vi "App_new_stream.vi"() -> ()   [LabVIEW 2015]
uses:
  <vilib>/DAQmx/read.llb/DAQmx Read (Analog Wfm 1Chan NSamp).vi
  <vilib>/DAQmx/miscellaneous.llb/DAQmx Fill In Error Info.vi
panel:
  in  "task out":refnum<k21>
  out "Button 2":u16
  out "Waveform Chart 2":waveform(dbl)
  out "Button":u16
  in  "Tab Control":T1(tab)
  out "min value":dbl
  out "max value":dbl
  out "Delta(s)":dbl
  in  "Zero":bool
  out "Average":dbl
  in  "mA/uA":bool
  out "Waveform Graph":waveform(dbl)(graph)
  in  "uA/mA":bool=TRUE
  out "Waveform Graph 2":waveform(dbl)(graph)
  out "Average (uA)":dbl
  in  "PAUSE":bool
  out "Vbat":dbl
  out "Waveform Chart":dbl(graph)
  in  "Number of samples uC Board":i32=10000
  in  "USB DAQ":tag="Dev1"
  out "Waveform Chart 3":dbl(graph)
  in  "file List":i32(listbox)
  out "2D Picture":picture
  # "FW Validation - Current Tracking V1.0"
  # "For uC Board: 20kS/s"
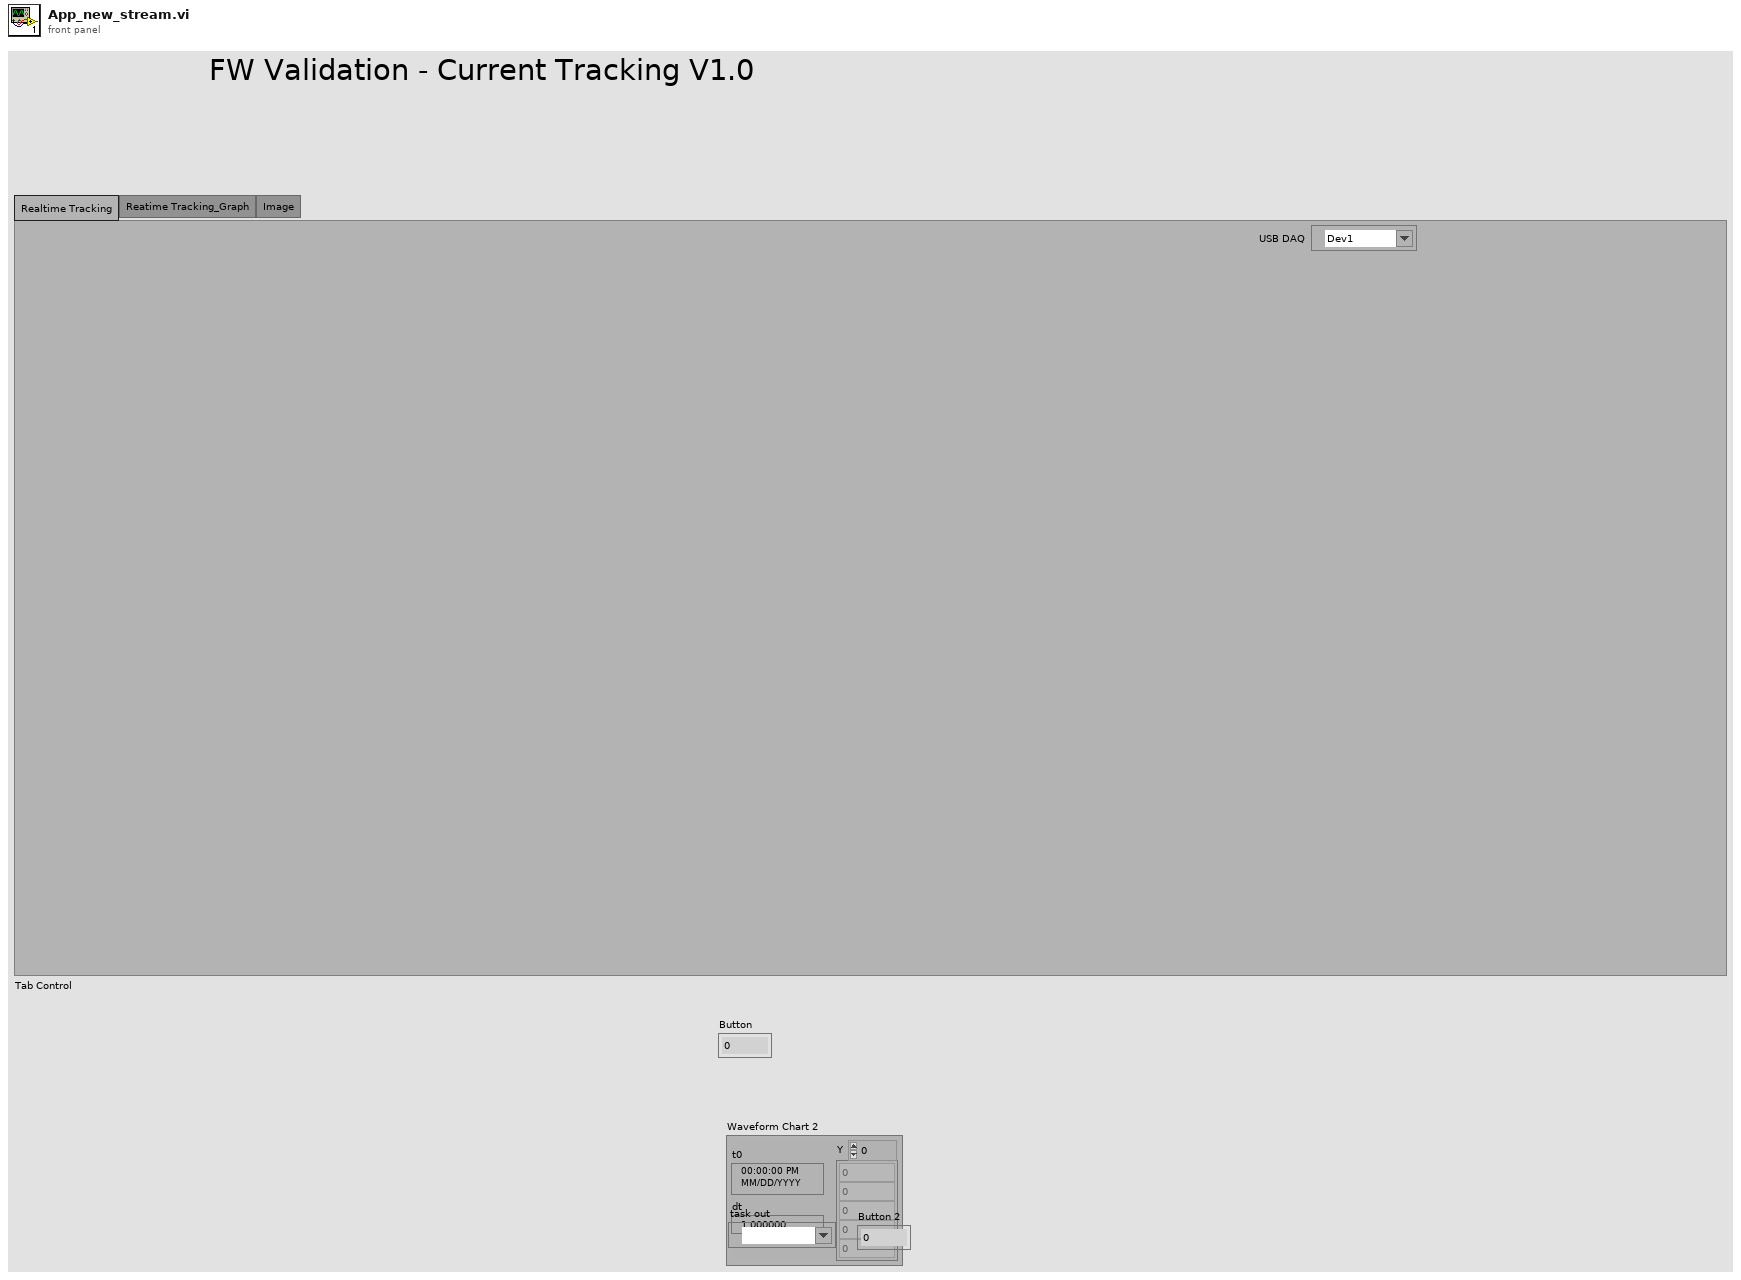
[diagram p1: front panel]
types:
  T1 = enum32{"Realtime Tracking", "Reatime Tracking_Graph", "Image"}
  T2 = typedef "imagedata.ctl" = cluster{"image type":i32, "image depth":i32, "image":u8[], "mask":u8[], "colors":u32[], "Rectangle":cluster{"left":i16, "top":i16, "right":i16, "bottom":i16}}
  T3 = typedef "LVCursorListTypeDef.ctl" = cluster{"Name":string, "Color":u32, "Style":u8, "Point Style":u8, "Name Visible":bool, "Allow Drag":bool, "Cursor Mode":u32, "Plot":i32, "Index":i32, "Position":cluster{"X":dbl, "Y":dbl}, "X Scale":u32, "Y Scale":u32, "Watch Plots":i32[], "Watch All Plots":bool, "Plot Area":i32, "Label Offset":cluster{"X":dbl, "Y":dbl}}[]
  T4 = cluster{"Name":string, "Color":u32, "Style":u8, "Point Style":u8, "Name Visible":bool, "Allow Drag":bool, "Cursor Mode":u32, "Plot":i32, "Index":i32, "Position":cluster{"X":dbl, "Y":dbl}, "X Scale":u32, "Y Scale":u32, "Watch Plots":i32[], "Watch All Plots":bool, "Plot Area":i32, "Label Offset":cluster{"X":dbl, "Y":dbl}}
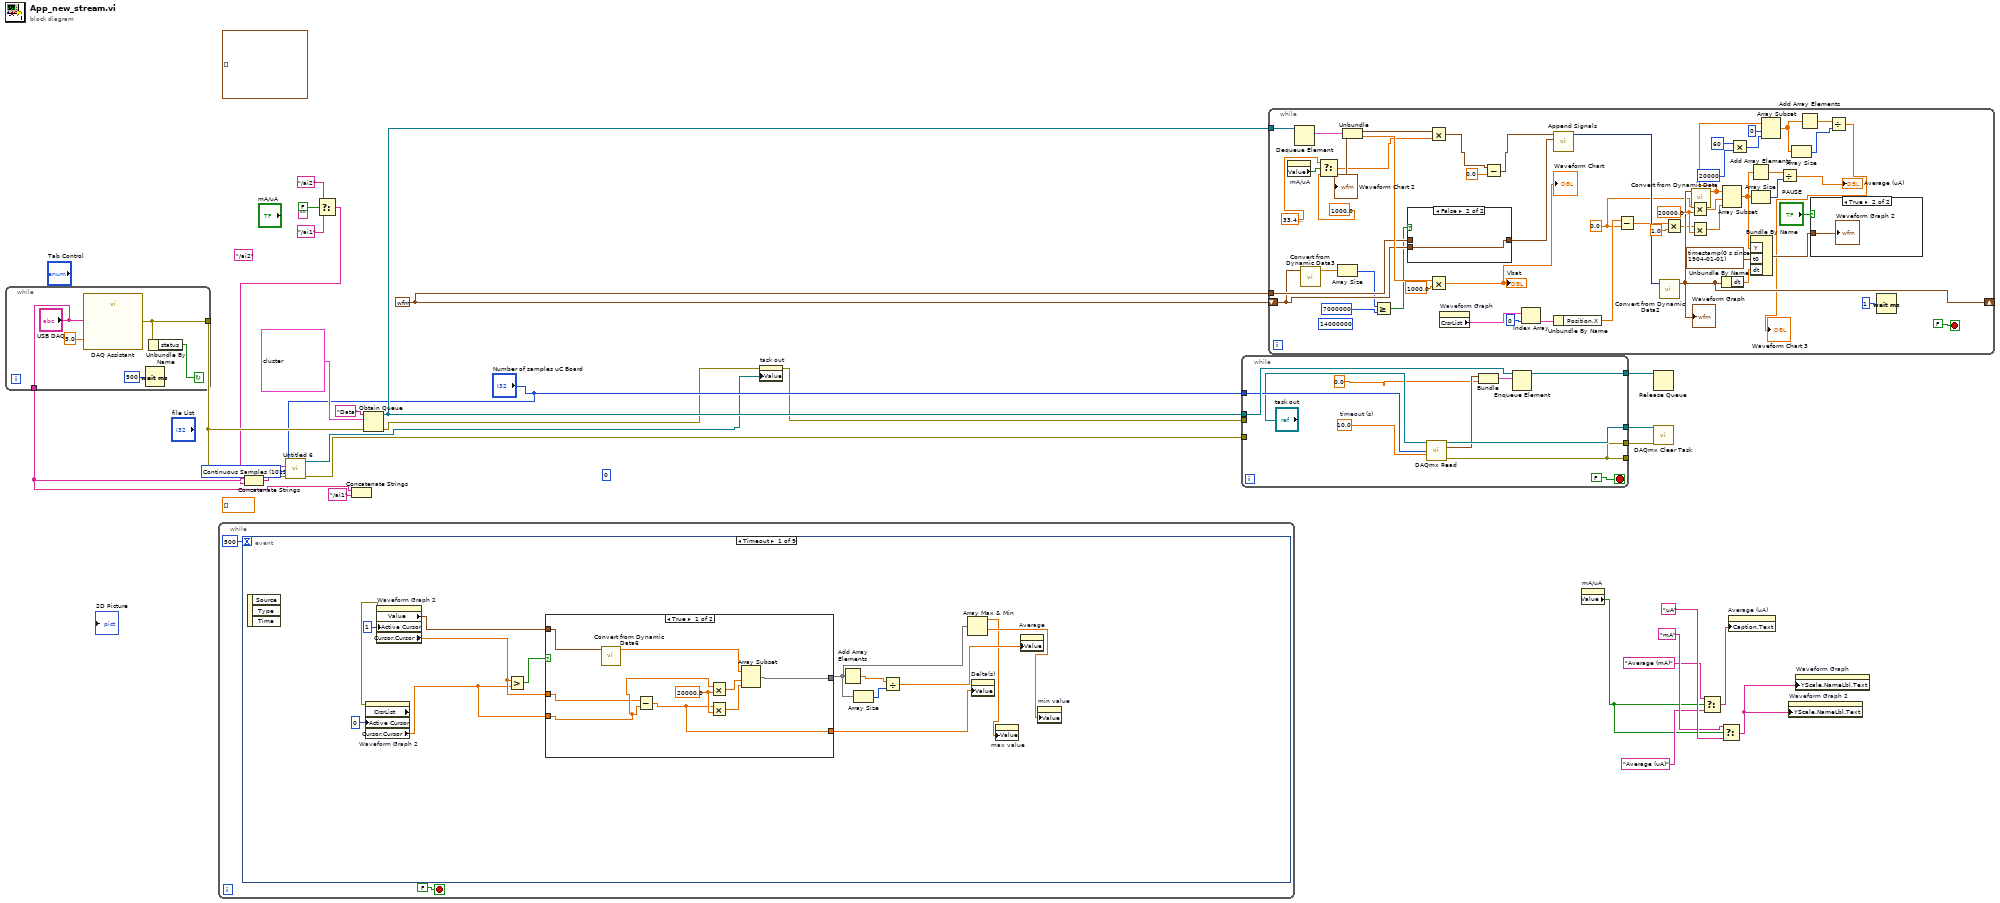
[diagram p0: block diagram]
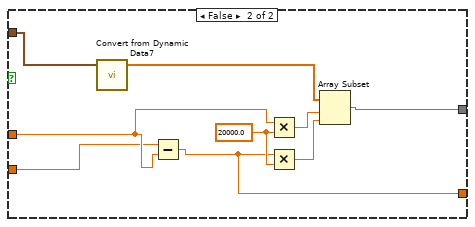
[diagram p2: hidden frame]
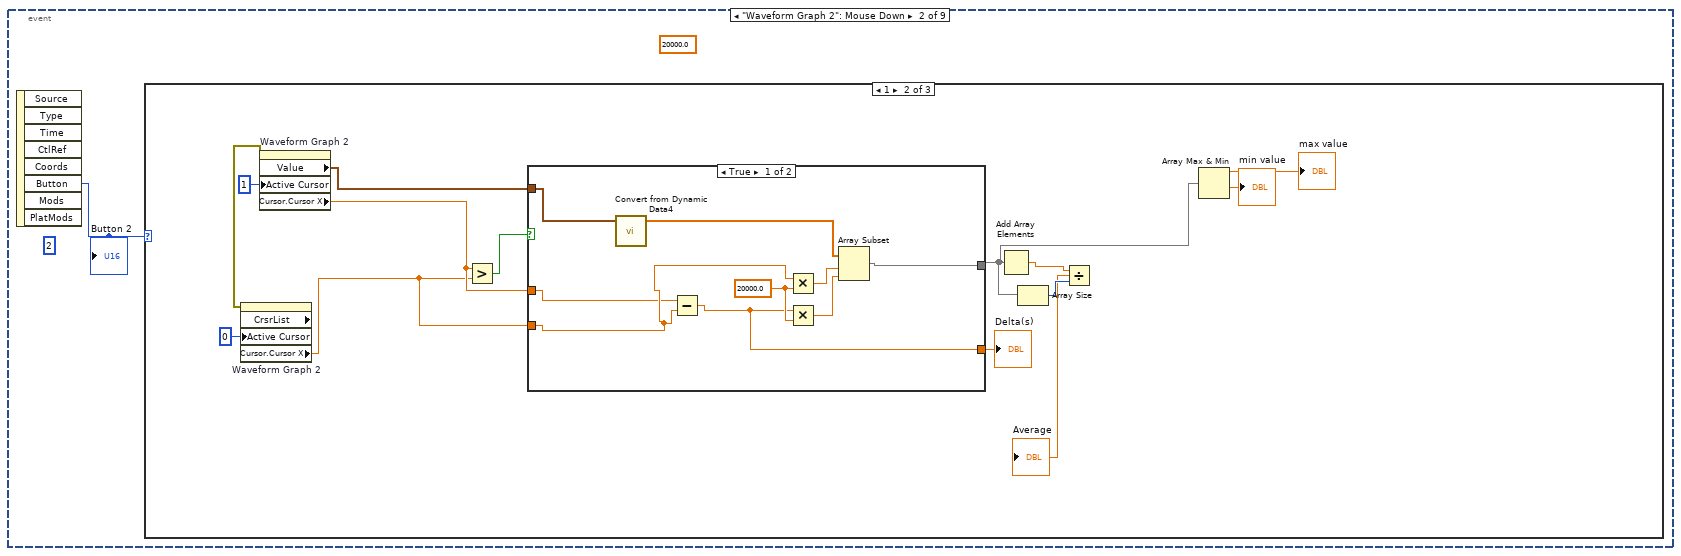
[diagram p3: hidden frame]
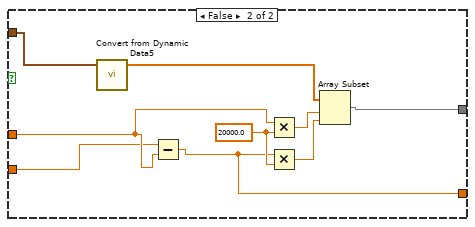
[diagram p5: hidden frame]
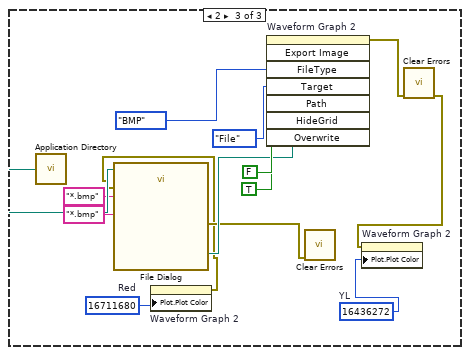
[diagram p6: hidden frame]
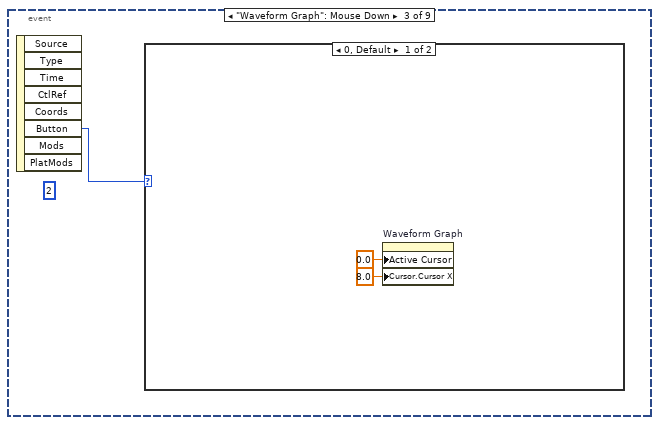
[diagram p7: hidden frame]
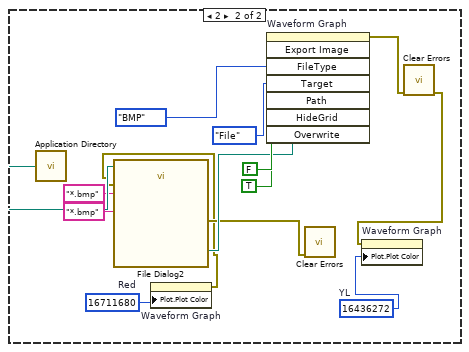
[diagram p8: hidden frame]
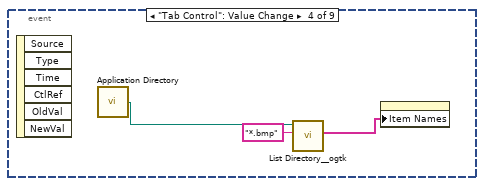
[diagram p9: hidden frame]
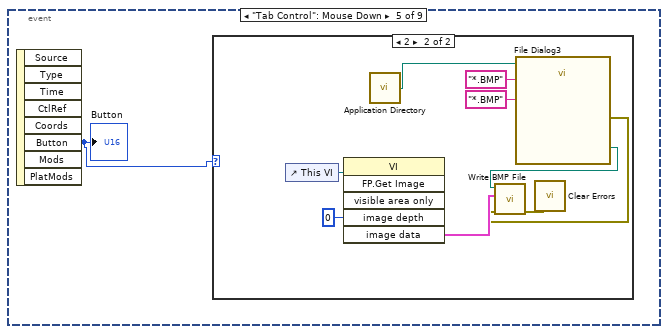
[diagram p10: hidden frame]
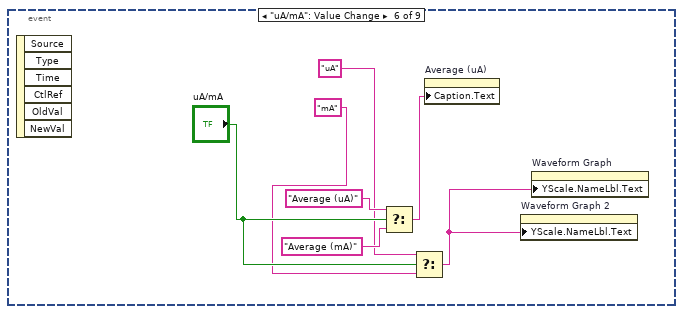
[diagram p12: hidden frame]
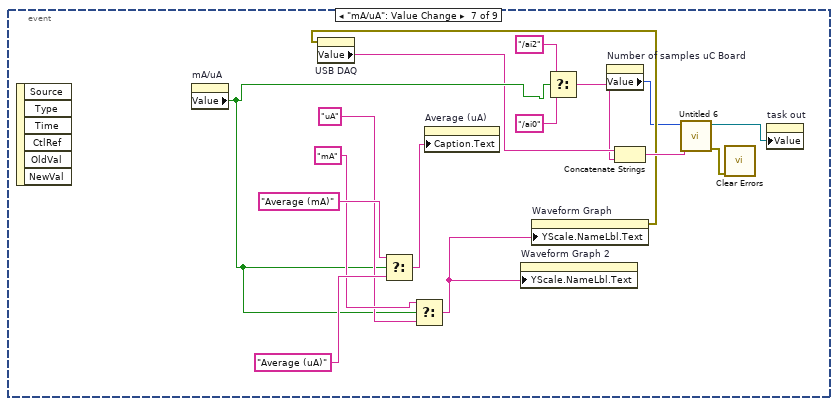
[diagram p13: hidden frame]
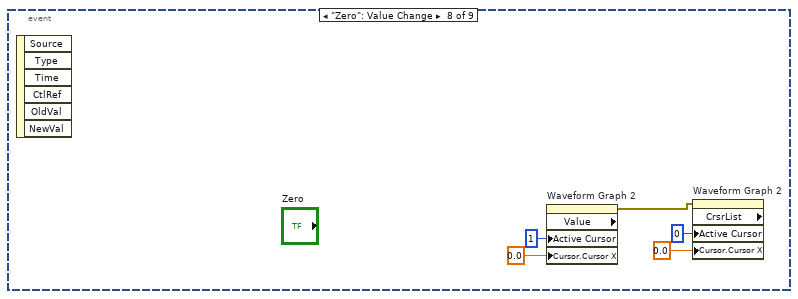
[diagram p14: hidden frame]
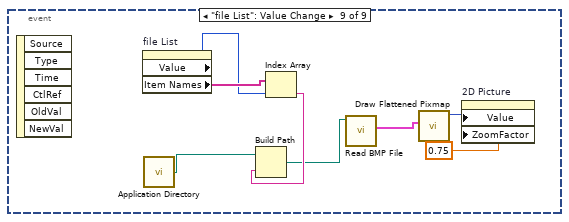
[diagram p15: hidden frame]
diagram:
  (unwired) "" ("f")
  w2 = 10123 items=["Finite Samples"=10178, "Continuous Samples"=10123, "Hardware Timed Single Point"=12522] ("sample mode")
  (unwired) u32 0 ("Active Cursor")
  (unwired) "/ai2" ("string")
  w20 = waveform(dbl) {"t0"=timestamp(0 s since 1904-01-01), "dt"=0.0, "Y"=[]} ("data")
  (unwired) waveform(dbl)[] [] ("History Data")
  (unwired) dbl[] [] ("Array")
  n1 = while {
    tunnel: [w31] -> w23
    tunnel: ["USB DAQ"] -> w17
    stop <- w30 continue-if-true
    n2 = call "DAQ Assistant"("data"=5.0, "device name"="USB DAQ") -> ("error out"=w31:errorcluster)  [unwired: 16 in, 1 out]
    n3 = Wait (ms)(milliseconds to wait=u32 500) -> ()  [unwired: 1 out]
    n4 = Unbundle By Name(w31) -> ("status"=w30:bool)
  }
  n5 = while {
    stop <- FALSE stop-if-true
    n6 = event shown="[0] Timeout" {
      selector: _ -> [_ _ _ _ _ _ _ _ _]
      dyn-events: _ -> [_ _ _ _ _ _ _ _ _]
      timeout: 500 -> [_ _ _ _ _ _ _ _ _]
      event Timeout {
        n7 = event-data() -> ()  [unwired: 1 in, 3 out]
        n8 = property on="Waveform Graph 2" class="WFGraph (strict)"("Active Cursor"=u32 1) -> (error out=w44:errorcluster, "Value"=w40:waveform(dbl), "Cursor.Cursor X"=w46:dbl)  [unwired: 2 in, 1 out]
        n9 = property on="Waveform Graph 2" class="WFGraph (strict)" props=["CrsrList", "Active Cursor", "Cursor", "Cursor X"](error in=w44, "Active Cursor"=u32 0) -> ("Cursor.Cursor X"=w45:dbl)  [unwired: 1 in, 3 out]
        n10 = Greater?(x=w46, y=w45) -> (0:w47:bool)
        n11 = case shown="True" w47 {
          tunnel: w40 -> [w58 w67]
          tunnel: w46 -> [w51 w61]
          tunnel: w45 -> [w52 w60]
          tunnel: [w53 w62] -> w41
          tunnel: [w50 w59] -> w39
          frame True {
            w56 = 20000.0 ("y")
            n12 = call "Convert from Dynamic Data6"("Dynamic Data Type"=w58) -> ("Array"=w54:dbl[])  [unwired: 3 in]
            n13 = Subtract(x=w51, y=w52) -> (x-y=w50:dbl)
            n14 = Multiply(x=w52, y=w56) -> (x*y=w57:dbl)
            n15 = Multiply(x=w50, y=w56) -> (x*y=w55:dbl)
            n16 = Array Subset(array=w54, index=w57, length=w55) -> (w53:dbl[])
          }
          frame False {
            w65 = 20000.0 ("y")
            n17 = call "Convert from Dynamic Data7"("Dynamic Data Type"=w67) -> ("Array"=w63:dbl[])  [unwired: 3 in]
            n18 = Subtract(x=w60, y=w61) -> (x-y=w59:dbl)
            n19 = Multiply(x=w61, y=w65) -> (x*y=w66:dbl)
            n20 = Multiply(x=w59, y=w65) -> (x*y=w64:dbl)
            n21 = Array Subset(array=w63, index=w66, length=w64) -> (w62:dbl[])
          }
        }
        n22 = Add Array Elements(numeric array=w41) -> (sum=w43:dbl)
        n23 = Array Size(array=w41) -> (size(s)=w42:i32)
        n24 = Divide(x=w43, y=w42) -> (x/y=w38:dbl)
        n25 = Array Max & Min(array=w41) -> (max value=w36:dbl, min value=w37:dbl)  [unwired: 2 out]
        n26 = property on="Delta(s)" class="DigNum (strict)"("Value"=w39) -> ()  [unwired: 2 in, 2 out]
        n27 = property on="max value" class="DigNum (strict)"("Value"=w36) -> ()  [unwired: 2 in, 2 out]
        n28 = property on="Average" class="DigNum (strict)"("Value"=w38) -> ()  [unwired: 2 in, 2 out]
        n29 = property on="min value" class="DigNum (strict)"("Value"=w37) -> ()  [unwired: 2 in, 2 out]
      }
      event "Waveform Graph 2": Mouse Down {
        (unwired) 20000.0 ("y")
        (unwired) u16 2 ("Button")
        n30 = event-data() -> ("Button"=w68:u16)  [unwired: 1 in, 7 out]
        "Button 2" <- w68
        n31 = case shown="1" w68 {
          frame 0, Default {
          }
          frame 1 {
            n32 = property on="Waveform Graph 2" class="WFGraph (strict)"("Active Cursor"=u32 1) -> (error out=w77:errorcluster, "Value"=w69:waveform(dbl), "Cursor.Cursor X"=w79:dbl)  [unwired: 2 in, 1 out]
            n33 = property on="Waveform Graph 2" class="WFGraph (strict)" props=["CrsrList", "Active Cursor", "Cursor", "Cursor X"](error in=w77, "Active Cursor"=u32 0) -> ("Cursor.Cursor X"=w78:dbl)  [unwired: 1 in, 3 out]
            n34 = Greater?(x=w79, y=w78) -> (0:w80:bool)
            n35 = case shown="True" w80 {
              tunnel: w69 -> [w91 w100]
              tunnel: w79 -> [w84 w94]
              tunnel: w78 -> [w85 w93]
              tunnel: [w86 w95] -> w72
              tunnel: [w83 w92] -> w73
              frame True {
                w89 = 20000.0 ("y")
                n36 = call "Convert from Dynamic Data4"("Dynamic Data Type"=w91) -> ("Array"=w87:dbl[])  [unwired: 3 in]
                n37 = Subtract(x=w84, y=w85) -> (x-y=w83:dbl)
                n38 = Multiply(x=w85, y=w89) -> (x*y=w90:dbl)
                n39 = Multiply(x=w83, y=w89) -> (x*y=w88:dbl)
                n40 = Array Subset(array=w87, index=w90, length=w88) -> (w86:dbl[])
              }
              frame False {
                w98 = 20000.0 ("y")
                n41 = call "Convert from Dynamic Data5"("Dynamic Data Type"=w100) -> ("Array"=w96:dbl[])  [unwired: 3 in]
                n42 = Subtract(x=w93, y=w94) -> (x-y=w92:dbl)
                n43 = Multiply(x=w94, y=w98) -> (x*y=w99:dbl)
                n44 = Multiply(x=w92, y=w98) -> (x*y=w97:dbl)
                n45 = Array Subset(array=w96, index=w99, length=w97) -> (w95:dbl[])
              }
            }
            "Delta(s)" <- w73
            n46 = Add Array Elements(numeric array=w72) -> (sum=w76:dbl)
            n47 = Array Size(array=w72) -> (size(s)=w75:i32)
            n48 = Divide(x=w76, y=w75) -> (x/y=→"Average":dbl)
            n49 = Array Max & Min(array=w72) -> (max value=→"max value":dbl, min value=→"min value":dbl)  [unwired: 2 out]
          }
          frame 2 {
            w101 = u32 16436272  # YL
            w103 = u32 16711680  # Red
            n50 = call <vilib>:"Application Directory.vi"() -> ("Application Directory"=w110:path)
            n51 = property on="Waveform Graph 2" class="WFGraph (strict)"("Plot.Plot Color"=w103) -> (error out=w104:errorcluster)  [unwired: 2 in, 1 out]
            n52 = call "File Dialog"("start path"=w110, "error in"=w104, "pattern (all files)"="*.bmp", "pattern label"="*.bmp") -> ("selected path"=w107:path, "error out"=w106:errorcluster)  [unwired: 8 in, 2 out]
            n53 = invoke on="Waveform Graph 2" class="WFGraph (strict)" method="Export Image"("FileType"=enum32{"BMP", "EPS", "EMF", "PICT"}."BMP" ("File Type"), "Target"=enum32{"File", "Clipboard"}."File", "Path"=w107, "HideGrid"=FALSE ("Hide Grid"), "Overwrite"=TRUE ("Always Overwrite")) -> (error out=w105:errorcluster)  [unwired: 3 in, 7 out]
            n54 = call <vilib>:"Clear Errors.vi"("error in (no error)"=w106) -> ()  [unwired: 5 in, 2 out]
            n55 = call <vilib>:"Clear Errors.vi"("error in (no error)"=w105) -> ("error out"=w102:errorcluster)  [unwired: 5 in, 1 out]
            n56 = property on="Waveform Graph 2" class="WFGraph (strict)"(error in=w102, "Plot.Plot Color"=w101) -> ()  [unwired: 1 in, 2 out]
          }
        }
      }
      event "Waveform Graph": Mouse Down {
        (unwired) u16 2 ("Button")
        n57 = event-data() -> ("Button"=w115:u16)  [unwired: 1 in, 7 out]
        n58 = case shown="0, Default" w115 {
          frame 0, Default {
            n59 = property on="Waveform Graph" class="WFGraph (strict)"("Active Cursor"=0.0 ("Cursor.Cursor Position:Cursor X"), "Cursor.Cursor X"=8.0 ("Cursor.Cursor Position:Cursor X")) -> ()  [unwired: 2 in, 2 out]
          }
          frame 2 {
            w118 = u32 16436272  # YL
            w120 = u32 16711680  # Red
            n60 = call <vilib>:"Application Directory.vi"() -> ("Application Directory"=w127:path)
            n61 = property on="Waveform Graph" class="WFGraph (strict)"("Plot.Plot Color"=w120) -> (error out=w121:errorcluster)  [unwired: 2 in, 1 out]
            n62 = call "File Dialog2"("start path"=w127, "error in"=w121, "pattern (all files)"="*.bmp", "pattern label"="*.bmp") -> ("selected path"=w124:path, "error out"=w123:errorcluster)  [unwired: 8 in, 2 out]
            n63 = invoke on="Waveform Graph" class="WFGraph (strict)" method="Export Image"("FileType"=enum32{"BMP", "EPS", "EMF", "PICT"}."BMP" ("File Type"), "Target"=enum32{"File", "Clipboard"}."File", "Path"=w124, "HideGrid"=FALSE ("Hide Grid"), "Overwrite"=TRUE ("Always Overwrite")) -> (error out=w122:errorcluster)  [unwired: 3 in, 7 out]
            n64 = call <vilib>:"Clear Errors.vi"("error in (no error)"=w123) -> ()  [unwired: 5 in, 2 out]
            n65 = call <vilib>:"Clear Errors.vi"("error in (no error)"=w122) -> ("error out"=w119:errorcluster)  [unwired: 5 in, 1 out]
            n66 = property on="Waveform Graph" class="WFGraph (strict)"(error in=w119, "Plot.Plot Color"=w118) -> ()  [unwired: 1 in, 2 out]
          }
        }
      }
      event "Tab Control": Value Change {
        n67 = event-data() -> ()  [unwired: 1 in, 6 out]
        n68 = call <vilib>:"Application Directory.vi"() -> ("Application Directory"=w134:path)
        n69 = call <userlib>:"List Directory__ogtk.vi"("pattern"="*.bmp", "directory path"=w134) -> ("file names"=w132:string[])  [unwired: 2 in, 3 out]
        n70 = property on="file List" class="LstBox (strict)"("Item Names"=w132) -> ()  [unwired: 2 in, 2 out]
      }
      event "Tab Control": Mouse Down {
        n71 = event-data() -> ("Button"=w135:u16)  [unwired: 1 in, 7 out]
        "Button" <- w135
        n72 = case shown="2" w135 {
          frame 0, Default {
          }
          frame 2 {
            n73 = control-ref of="This VI"() -> (w144:refnum<vi>)
            n74 = invoke class="VI" method="FP.Get Image"(reference=w144, "image depth"=0 ("Image Depth")) -> ("image data"=w142:T2)  [unwired: 4 in, 5 out]
            n75 = call <vilib>:"Application Directory.vi"() -> ("Application Directory"=w138:path)
            n76 = call "File Dialog3"("start path"=w138, "pattern (all files)"="*.BMP", "pattern label"="*.BMP") -> ("selected path"=w141:path, "error out"=w140:errorcluster)  [unwired: 9 in, 2 out]
            n77 = call <vilib>:"Write BMP File.vi"("error in (no error)"=w140, "image data"=w142, "path to BMP file"=w141) -> ("error out"=w136:errorcluster)  [unwired: 7 in, 1 out]
            n78 = call <vilib>:"Clear Errors.vi"("error in (no error)"=w136) -> ()  [unwired: 5 in, 2 out]
          }
        }
      }
      event "uA/mA": Value Change {
        n79 = event-data() -> ()  [unwired: 1 in, 6 out]
        n80 = Select(t="Average (uA)" ("Caption.Text"), s="uA/mA", f="Average (mA)" ("Caption.Text")) -> (s? t:f=w151:string)
        n81 = Select(t="uA" ("Caption.Text"), s="uA/mA", f="mA" ("Caption.Text")) -> (s? t:f=w145:string)
        n82 = property on="Average (uA)" class="DigNum (strict)"("Caption.Text"=w151) -> ()  [unwired: 2 in, 2 out]
        n83 = property on="Waveform Graph 2" class="WFGraph (strict)"("YScale.NameLbl.Text"=w145) -> ()  [unwired: 2 in, 2 out]
        n84 = property on="Waveform Graph" class="WFGraph (strict)"("YScale.NameLbl.Text"=w145) -> ()  [unwired: 2 in, 2 out]
      }
      event "mA/uA": Value Change {
        n85 = event-data() -> ()  [unwired: 1 in, 6 out]
        n86 = property on="mA/uA" class="Bool (strict)"() -> ("Value"=w159:bool)  [unwired: 2 in, 2 out]
        n87 = Select(t="Average (mA)" ("Caption.Text"), s=w159, f="Average (uA)" ("Caption.Text")) -> (s? t:f=w167:string)
        n88 = Select(t="mA" ("Caption.Text"), s=w159, f="uA" ("Caption.Text")) -> (s? t:f=w166:string)
        n89 = property on="Average (uA)" class="DigNum (strict)"("Caption.Text"=w167) -> ()  [unwired: 2 in, 2 out]
        n90 = property on="Waveform Graph 2" class="WFGraph (strict)"("YScale.NameLbl.Text"=w166) -> ()  [unwired: 2 in, 2 out]
        n91 = property on="Waveform Graph" class="WFGraph (strict)"("YScale.NameLbl.Text"=w166) -> (error out=w155:errorcluster)  [unwired: 2 in, 1 out]
        n92 = property on="USB DAQ" class="DAQmxName"(error in=w155) -> ("Value"=w157:string)  [unwired: 1 in, 2 out]
        n93 = Select(t="/ai2" ("string"), s=w159, f="/ai0" ("string")) -> (s? t:f=w156:string)
        n94 = property on="Number of samples uC Board" class="DigNum (strict)"() -> ("Value"=w154:i32)  [unwired: 2 in, 2 out]
        n95 = Concatenate Strings(w157, w156) -> (w158:string)
        n96 = call "Untitled 6.vi"("physical channel"=w158, "number of samples"=w154) -> ("error out"=w152:errorcluster, "task out"=w153:refnum<k21>)  [unwired: 8 in]
        n97 = call <vilib>:"Clear Errors.vi"("error in (no error)"=w152) -> ()  [unwired: 5 in, 2 out]
        n98 = property on="task out" class="DAQmxName (strict)"("Value"=w153) -> ()  [unwired: 2 in, 2 out]
      }
      event "Zero": Value Change {
        n99 = event-data() -> ()  [unwired: 1 in, 6 out]
        n100 = property on="Waveform Graph 2" class="WFGraph (strict)" props=["Value", "Active Cursor", "Cursor", "Cursor X"]("Active Cursor"=u32 1, "Cursor.Cursor X"=0.0 ("Cursor.Cursor Position:Cursor X")) -> (error out=w170:errorcluster)  [unwired: 2 in, 2 out]
        n101 = property on="Waveform Graph 2" class="WFGraph (strict)" props=["CrsrList", "Active Cursor", "Cursor", "Cursor X"](error in=w170, "Active Cursor"=u32 0, "Cursor.Cursor X"=0.0 ("Cursor.Cursor Position:Cursor X")) -> ()  [unwired: 1 in, 3 out]
      }
      event "file List": Value Change {
        n102 = event-data() -> ()  [unwired: 1 in, 6 out]
        n103 = property on="file List" class="LstBox (strict)"() -> ("Value"=w179:i32, "Item Names"=w180:string[])  [unwired: 2 in, 2 out]
        n104 = call <vilib>:"Application Directory.vi"() -> ("Application Directory"=w176:path)
        n105 = Index Array(array=w180, index=w179) -> (element=w175:string)
        n106 = Build Path(base path=w176, name or relative path=w175) -> (appended path=w174:path)
        n107 = call <vilib>:"Read BMP File.vi"("path to BMP file"=w174) -> ("image data"=w178:T2)  [unwired: 8 in, 2 out]
        n108 = call <vilib>:"Draw Flattened Pixmap.vi"("image data"=w178) -> ("new picture"=w177:picture)  [unwired: 8 in]
        n109 = property on="2D Picture" class="Pict"("Value"=w177, "ZoomFactor"=sgl 0.75 ("Zoom Factor")) -> ()  [unwired: 2 in, 2 out]
      }
    }
  }
  n110 = Select(t="/ai2" ("string"), s=FALSE, f="/ai1" ("string")) -> (s? t:f=w13:string)
  n111 = Concatenate Strings(w17, w13) -> (w18:string)
  n112 = call "Untitled 6.vi"("error in"=w23, "sample mode"=w2, "physical channel"=w18, "number of samples"="Number of samples uC Board") -> ("error out"=w22:errorcluster, "task out"=w5:refnum<k21>)  [unwired: 6 in]
  n113 = Concatenate Strings(w17, "/ai1" ("string")) -> ()  [unwired: 1 out]
  n114 = Obtain Queue(name (unnamed)="Data", element data type=cluster{"Waveform Chart 2":waveform(dbl), dbl} {"Waveform Chart 2"={"t0"=timestamp(0 s since 1904-01-01), "dt"=1.0, "Y"=[]}, 0.0}, error in (no error)=w23) -> (queue out=w25:refnum<queue>, error out=w4:errorcluster)  [unwired: 2 in, 1 out]
  n115 = property on="task out" class="DAQmxName (strict)"(error in=w4, "Value"=w5) -> (error out=w3:errorcluster)  [unwired: 1 in, 1 out]
  n116 = while {
    tunnel: w22 -> [_]
    tunnel: [w191] -> w28
    tunnel: [w186] -> w27
    tunnel: w25 -> [w189]
    tunnel: [w188] -> w24
    tunnel: [w186] -> _
    tunnel: "Number of samples uC Board" -> [w183]
    tunnel: w3 -> [_]
    stop <- FALSE ("stop (F)") stop-if-true
    w190 = 10.0  # timeout (s)
    n117 = call-poly <vilib>:"DAQmx Read.vi"("task/channels in"="task out", "number of samples per channel"=w183, "timeout"=w190) -> ("task out"=w191:refnum<k21>, "data"=w185:waveform(dbl), "error out"=w186:errorcluster)  [unwired: 10 in]
    n118 = Bundle("data"=w185, "data"=0.0) -> (w184:cluster{"data":waveform(dbl), "data":dbl})  [unwired: 1 in]
    n119 = Enqueue Element(queue=w189, element=w184) -> (queue out=w188:refnum<queue>)  [unwired: 2 in, 2 out]
  }
  n120 = while {
    tunnel: w25 -> [w243]
    shift-right: [w232] -> _
    shift-left: w20 -> [w212]
    tunnel: w20 -> [w213]
    stop <- FALSE stop-if-true
    (unwired) 14000000 ("size(s)")
    w222 = 0.0
    w236 = 20000.0 ("y")
    n121 = property on="mA/uA" class="Bool (strict)"() -> ("Value"=w204:bool)  [unwired: 2 in, 2 out]
    n122 = Dequeue Element(queue=w243) -> (element=w219:cluster{"Waveform Chart 2":waveform(dbl), dbl})  [unwired: 2 in, 3 out]
    n123 = call "Convert from Dynamic Data3"("Dynamic Data Type"=w212) -> ("Array"=w211:dbl[])  [unwired: 3 in]
    n124 = Select(t=33.499999999999986 ("y"), s=w204, f=1000.0 ("y")) -> (s? t:f=w201:dbl)
    n125 = Array Size(array=w211) -> (size(s)=w210:i32)
    n126 = Unbundle(w219) -> ("Waveform Chart 2"=w218:waveform(dbl), w217:dbl)
    "Waveform Chart 2" <- w218
    n127 = Greater Or Equal?(x=w210, y=7000000 ("size(s)")) -> (x >= y?=w208:bool)
    n128 = case shown="False" w208 {
      tunnel: w212 -> [_ w245]
      tunnel: [w244 w245] -> w214
      tunnel: w213 -> [w244 _]
      frame True {
      }
      frame False {
      }
    }
    n129 = Multiply(x=w218, y=w201) -> (x*y=w205:waveform(dbl))
    n130 = Multiply(x=w217, y=1000.0) -> (x*y=→"Vbat" →"Waveform Chart":dbl)
    n131 = property on="Waveform Graph" class="WFGraph (strict)"() -> ("CrsrList"=w239:T3)  [unwired: 2 in, 2 out]
    n132 = Subtract(x=w205, y=0.0) -> (x-y=w206:waveform(dbl))
    n133 = Index Array(array=w239, index=0) -> (element=w220:T4)
    n134 = call "Append Signals"("Input Signal B"=w214, "Input Signal A"=w206) -> ("Appended Signals"=w240:dynamicdata)  [unwired: 8 in, 1 out]
    n135 = Unbundle By Name(w220) -> ("Position.X"=w223:dbl)
    n136 = Subtract(x=w223, y=w222) -> (x-y=w226:dbl)
    n137 = call "Convert from Dynamic Data2"("Dynamic Data Type"=w240) -> ("Waveform"=w232:waveform(dbl))  [unwired: 3 in]
    "Waveform Graph" <- w232
    n138 = Multiply(x=w226, y=1.0) -> (x*y=w224:dbl)
    n139 = Multiply(x=w222, y=w236) -> (x*y=w237:dbl)
    n140 = Multiply(x=w224, y=w236) -> (x*y=w235:dbl)
    n141 = call "Convert from Dynamic Data"("Dynamic Data Type"=w232) -> ("Array"=w199:dbl[])  [unwired: 3 in]
    n142 = Unbundle By Name(w232) -> ("dt"=w231:dbl)
    n143 = Array Subset(array=w199, index=w237, length=w235) -> (w230:dbl[])
    n144 = Multiply(x=60, y=20000) -> (x*y=w195:i32)
    n145 = Add Array Elements(numeric array=w230) -> (sum=w229:dbl)
    n146 = Bundle By Name("Y"=w230, "t0"=timestamp(0 s since 1904-01-01), "dt"=w231) -> (w234:waveform(dbl))  [unwired: 1 in]
    n147 = Array Size(array=w230) -> (size(s)=w228:i32)
    n148 = Array Subset(array=w199, index=0, length=w195) -> (w198:dbl[])
    n149 = Divide(x=w229, y=w228) -> (x/y=→"Average (uA)":dbl)
    n150 = Array Size(array=w198) -> (size(s)=w197:i32)
    n151 = Add Array Elements(numeric array=w198) -> (sum=w200:dbl)
    n152 = case shown="True" "PAUSE" {
      tunnel: w234 -> [_ w246]
      frame False {
      }
      frame True {
        "Waveform Graph 2" <- w246
      }
    }
    n153 = Divide(x=w200, y=w197) -> (x/y=→"Waveform Chart 3":dbl)
    n154 = Wait (ms)(milliseconds to wait=u32 1) -> ()  [unwired: 1 out]
  }
  n155 = property on="mA/uA" class="Bool (strict)"() -> ("Value"=w8:bool)  [unwired: 2 in, 2 out]
  n156 = Release Queue(queue=w24) -> ()  [unwired: 2 in, 3 out]
  n157 = call <vilib>:"DAQmx Clear Task.vi"("task in"=w28, "error in"=w27) -> ()  [unwired: 13 in, 1 out]
  n158 = Select(t="Average (mA)" ("Caption.Text"), s=w8, f="Average (uA)" ("Caption.Text")) -> (s? t:f=w6:string)
  n159 = Select(t="mA" ("Caption.Text"), s=w8, f="uA" ("Caption.Text")) -> (s? t:f=w7:string)
  n160 = property on="Average (uA)" class="DigNum (strict)"("Caption.Text"=w6) -> ()  [unwired: 2 in, 2 out]
  n161 = property on="Waveform Graph 2" class="WFGraph (strict)"("YScale.NameLbl.Text"=w7) -> ()  [unwired: 2 in, 2 out]
  n162 = property on="Waveform Graph" class="WFGraph (strict)"("YScale.NameLbl.Text"=w7) -> ()  [unwired: 2 in, 2 out]
